vi "Send HTTP (SubVI).vi"(8 "error in (no error)":errorcluster, 10 "Thingworx Server Information":T1, 11 "Refnum in":T2) -> (0 "error out":errorcluster, 1 "Application Key":string, 2 "headers":string, 3 "Refnum out":T2, 4 "Complete Request URL":string, 5 "body":string)   [LabVIEW 2018]
uses:
  <vilib>/httpClient/ClientHandle.ctl
  <vilib>/httpClient/POSTBuffer.vi
  <vilib>/httpClient/PUTBuffer.vi
  <vilib>/httpClient/LabVIEWHTTPClient.lvlib
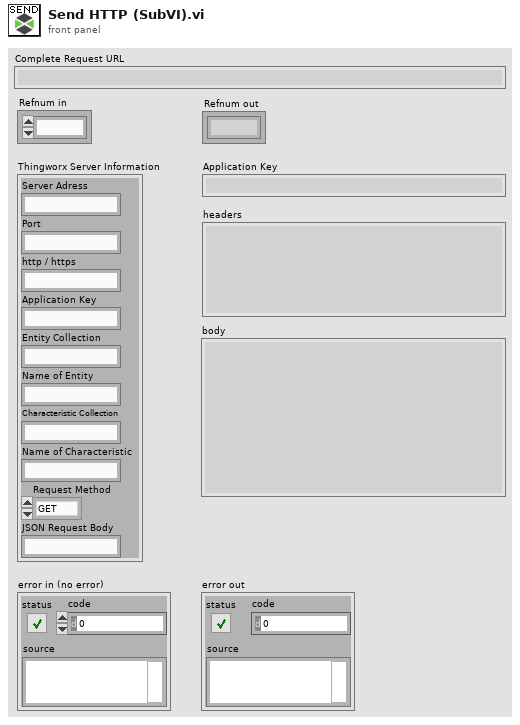
[diagram p1: front panel]
types:
  T1 = cluster{"Server Adress":string, "Port":string, "http / https":string, "Application Key":string, "Entity Collection":string, "Name of Entity":string, "Characteristic Collection":string, "Name of Characteristic":string, "Request Method":enum32{"GET", "POST", "DELETE", "PUT"}, "JSON Request Body":string}
  T2 = typedef "LabVIEWHTTPClient.lvlib/ClientHandle.ctl" = refnum<k1>
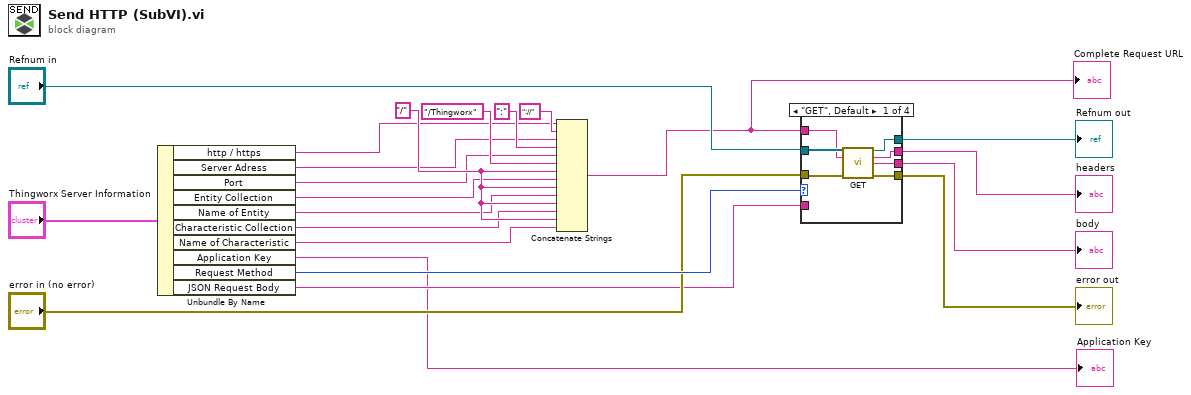
[diagram p0: block diagram]
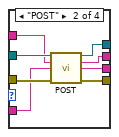
[diagram p2: hidden frame]
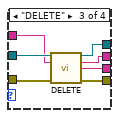
[diagram p3: hidden frame]
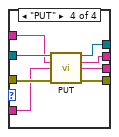
[diagram p4: hidden frame]
diagram:
  w14 = "/" ("string")
  n1 = Unbundle By Name("Thingworx Server Information") -> ("http / https"=w3:string, "Server Adress"=w5:string, "Port"=w7:string, "Entity Collection"=w10:string, "Name of Entity"=w11:string, "Characteristic Collection"=w12:string, "Name of Characteristic"=w13:string, "Application Key"=→"Application Key":string, "Request Method"=w18:enum32{"GET", "POST", "DELETE", "PUT"}, "JSON Request Body"=w16:string)
  n2 = Concatenate Strings(w3, "://" ("string"), w5, ":" ("string"), w7, "/Thingworx" ("string"), w14, w10, w14, w11, w14, w12, w14, w13) -> (w1:string)
  "Complete Request URL" <- w1
  n3 = case shown="\"GET\", Default" w18 {
    tunnel: "Refnum in" -> [w29 w37 w44 w52]
    tunnel: "error in (no error)" -> [w28 w36 w43 w51]
    tunnel: w1 -> [w23 w31 w38 w46]
    tunnel: [w27 w35 w42 w50] -> w22
    tunnel: [w26 w34 w41 w49] -> w19
    tunnel: [w25 w33 w40 w48] -> w21
    tunnel: [w24 w32 w39 w47] -> w20
    tunnel: w16 -> [_ w30 _ w45]
    frame "GET", Default {
      n4 = call <vilib>:"GET.vi"("client handle"=w29, "url"=w23, "error in (no error)"=w28) -> ("client handle out"=w27:T2, "headers"=w24:string, "body"=w25:string, "error out"=w26:errorcluster)  [unwired: 9 in]
    }
    frame "POST" {
      n5 = call-poly <vilib>:"POST.vi"("client handle"=w37, "url"=w31, "buffer"=w30, "error in (no error)"=w36) -> ("client handle out"=w35:T2, "headers"=w32:string, "body"=w33:string, "error out"=w34:errorcluster)  [unwired: 8 in]
    }
    frame "DELETE" {
      n6 = call <vilib>:"DELETE.vi"("client handle"=w44, "url"=w38, "error in (no error)"=w43) -> ("client handle out"=w42:T2, "headers"=w39:string, "body"=w40:string, "error out"=w41:errorcluster)  [unwired: 9 in]
    }
    frame "PUT" {
      n7 = call-poly <vilib>:"PUT.vi"("client handle"=w52, "url"=w46, "buffer"=w45, "error in (no error)"=w51) -> ("client handle out"=w50:T2, "headers"=w47:string, "body"=w48:string, "error out"=w49:errorcluster)  [unwired: 8 in]
    }
  }
  "Refnum out" <- w22
  "body" <- w21
  "headers" <- w20
  "error out" <- w19
